vi "Extract Tip.vi"(6 "Label":string, 8 "error in (no error)":errorcluster, 9 "Tip Number":i32, 10 "Mouse Position":cluster{"X":i32, "Y":i32}, 11 "Image":T1) -> (0 "error out":errorcluster, 3 "Tip Image":T1)   [LabVIEW 2013]
uses:
  <vilib>/vision/Image Controls.llb/IMAQ Image.ctl
  <vilib>/vision/NI_Vision_Development_Module.lvlib
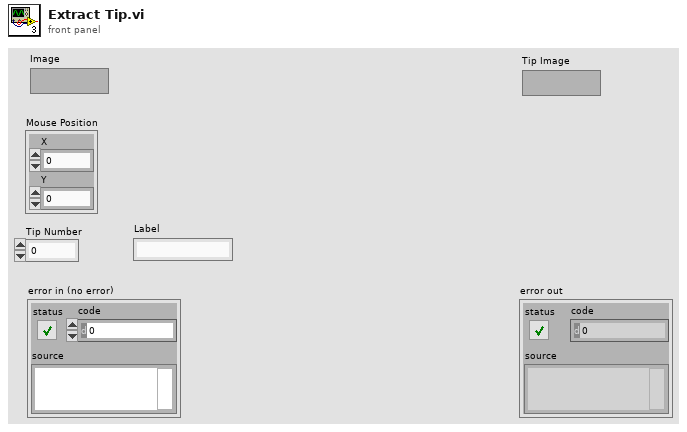
[diagram p1: front panel]
types:
  T1 = typedef "IMAQ Image.ctl" = refnum<image>
  T2 = cluster{"Left":i32, "Top":i32, "Right":i32, "Bottom":i32}
  T3 = typedef "Image Type" = u32
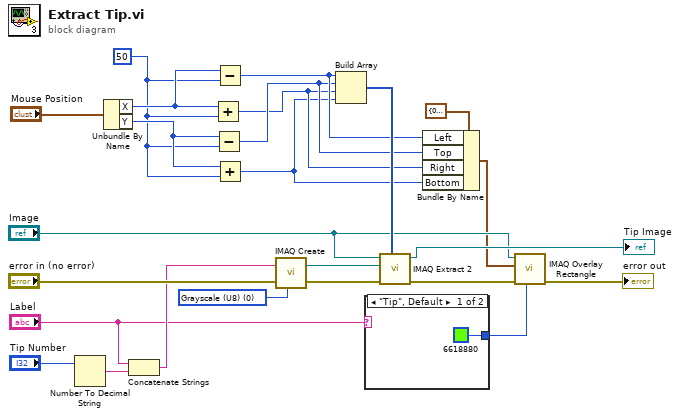
[diagram p0: block diagram]
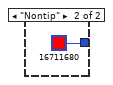
[diagram p2: hidden frame]
diagram:
  w13 = 50
  w20 = T3 0 items=["Grayscale (U8)", "Grayscale (I16)", "Grayscale (SGL)", "Complex (CSG)", "RGB (U32)", "HSL (U32)", "RGB (U64)", "Grayscale (U16)"] ("Image Type")
  n1 = Number To Decimal String(number="Tip Number") -> (decimal integer string=w22:string)  [unwired: 1 in]
  n2 = Unbundle By Name("Mouse Position") -> ("X"=w15:i32, "Y"=w14:i32)
  n3 = Concatenate Strings("Label", w22) -> (w21:string)
  n4 = Add(x=w15, y=w13) -> (x+y=w6:i32)
  n5 = Subtract(x=w14, y=w13) -> (x-y=w7:i32)
  n6 = Subtract(x=w15, y=w13) -> (x-y=w8:i32)
  n7 = Add(x=w14, y=w13) -> (x+y=w5:i32)
  n8 = call "IMAQ Create"("Image Name"=w21, "Image Type"=w20, "error in (no error)"="error in (no error)") -> ("New Image"=w18:T1, "error out"=w19:errorcluster)  [unwired: 2 in]
  n9 = Build Array(w8, w7, w6, w5) -> (w12:i32[])
  n10 = case shown="\"Tip\", Default" "Label" {
    tunnel: [u32 6618880 ("Color Box") u32 16711680 ("Color Box")] -> w2
    frame "Tip", Default {
    }
    frame "Nontip" {
    }
  }
  n11 = call "IMAQ Extract 2"("Optional Rectangle"=w12, "error in (no error)"=w19, "Image Dst"=w18, "Image Src"="Image") -> ("error out"=w11:errorcluster, "Image Dst Out"=→"Tip Image":T1)  [unwired: 6 in]
  n12 = Bundle By Name(cluster=T2 {"Left"=0, "Top"=0, "Right"=0, "Bottom"=0} ("Rectangle"), "Left"=w8, "Top"=w7, "Right"=w6, "Bottom"=w5) -> (w4:T2)
  n13 = call "IMAQ Overlay Rectangle"("Color"=w2, "error in (no error)"=w11, "Rectangle"=w4, "Image"="Image") -> ("error out"=→"error out":errorcluster)  [unwired: 6 in, 1 out]
